vi "Dashboard Main.vi"() -> ()   [LabVIEW 2012]
uses:
  <vilib>/event_ctls.llb/eventvkey.ctl
  <vilib>/Utility/config.llb/Read Key (String).vi
  <vilib>/Utility/config.llb/Read Key (I32).vi
  <vilib>/Utility/config.llb/Write Key (String).vi
  <vilib>/Utility/config.llb/Write Key (I32).vi
  <vilib>/Utility/config.llb/NI_LVConfig.lvlib
panel:
  out "Battery Value":dbl(slide) scale=0.0..14.0 scale format="%#_2e"
  out "Battery":sgl(graph)
  in  "Camera Settings":T1={"Frate Rate"=30, "Compression"=30, "Size"=1} {"Frate Rate" scale=1.0..30.0; "Size" items=["640x480", "320x240", "160x120"]}
  out "Mode":T2(ring)=enum."Auto Disabled"
  out "Camera IP":string
  out "JS1 Z":dbl(slide) scale=-1.0..1.0 scale format="%#_2e"
  out "JS2 Z":dbl(slide) scale=-1.0..1.0 scale format="%#_2e"
  out "Joystick 1":cluster{"X":dbl, "Y":dbl}[](graph)
  out "Joystick 2":cluster{"X":dbl, "Y":dbl}[](graph)
  out "JS Buttons 1":T3
  out "JS Buttons 2":T3
  out "MotorSlide4":dbl(slide) scale=-1.0..1.0 scale format="%#_2e"
  out "MotorSlide3":dbl(slide) scale=-1.0..1.0 scale format="%#_2e"
  out "MotorSlide2":dbl(slide) scale=-1.0..1.0 scale format="%#_2e"
  out "MotorName3":string="Front Left"
  out "MotorName4":string="Front Right"
  out "MotorName1":string="Rear Left"
  out "MotorName2":string="Rear Right"
  out "MotorChart4":dbl(graph)
  out "MotorChart3":dbl(graph)
  out "MotorChart2":dbl(graph)
  out "MotorSlide1":dbl(slide) scale=-1.0..1.0 scale format="%#_2e"
  out "MotorChart1":dbl(graph)
  out "Robot IP":string
  in  "Dashboard Tab":T4(tab)
  in  "Disable Autonomous":bool
  out "Arm Hook Sensor":bool
  out "Arm Encoder":dbl(knob) scale=0.0..100.0
  in  "notes":string
  out "Right Hook Sensor":bool
  out "Left Hook Sensor":bool
  out "Encoder Set":bool
  out "Arm Limit":bool
  in  "Y-Throttle":dbl(slide)=1.0 min=0.0 max=1.0 step=0.1 scale=0.0..1.0
  in  "X-Throttle":dbl(slide)=1.0 min=0.0 max=1.0 step=0.1 scale=0.0..1.0
  in  "Dev Notes":string
  in  "Robot Subsystems":enum32{"Drive", "Arm", "Sensors", "Hotkeys"}(tab)
  out "Left Wheel Encoder":dbl
  out "Right Wheel Encoder":dbl
  in  "Override Limit":bool
  out "Right Ultrasonic PWM":dbl(slide) scale=0.0..100.0
  out "Gyro":dbl(knob) scale=-180.0..180.0
  out "Left Ultrasonic PWM":dbl(slide) scale=0.0..100.0
  out "Hotkey Step":dbl
  out "Arm Preset":dbl
  in  "Current Hotkey":string
  out "Hotkey Running?":bool
  in  "Sim":bool=TRUE
  in  "Slider":dbl(slide) scale=0.0..100.0 scale format="%#_3g"
  in  "On/Off":bool caption="Solenoid"
  in  "Test Name":u16(ring) items=["Select the test to run...", "Example Test", "-------------------------------", "List of tests is built in robot code.", "Replace with your own automated tests."]
  in  "Test Tree":string(tree)
  in  "Motor":cluster{"Value":dbl, "Enable":bool} {"Value" scale=-1.0..1.0 scale format="%#_3g"}
  out "Progress":T5 {"Test Progress" scale=0.0..100.0}
  in  "Rev/Fwd":cluster{"Forward":bool, "Reverse":bool}
  in  "Ring":u16(ring) items=["Auto", "Fixed indoor", "Fixed outdoor 1", "Fixed outdoor 2", "Fixed fluorescent 1", "Fixed fluorescent 2", "Hold current"]
  in  "Listbox":i32(listbox)
  in  "Viewer":T6(tab)
  out "Mbps":dbl format="%#.1g"
  in  "Enable":bool
  in  "DB Camera Config":bool
  out "Mbps":bool
  out "fps":dbl format="%#.1g"
  out "Image Error Message":string="Timeout in Camera Communications"
  out "Camera Image":T7(plugin-control)
  out "Buttons 1":cluster{"1":bool, "2":bool, "3":bool}
  out "Kinect 1":cluster{"X":dbl, "Y":dbl, "Z":dbl} {"X" scale=1.0..-1.0; "Y" scale=1.0..-1.0; "Z" scale=1.0..-1.0}
  out "Buttons 2":cluster{"1":bool, "2":bool, "3":bool}
  out "Kinect 2":cluster{"X":dbl, "Y":dbl, "Z":dbl} {"X" scale=1.0..-1.0; "Y" scale=1.0..-1.0; "Z" scale=1.0..-1.0}
  out "Version":string
  out "Skeleton Picture":picture
  out "Players":i8
  out "Tree":string(tree)
  # "Drive & Motors"
  # "Robot IP:"
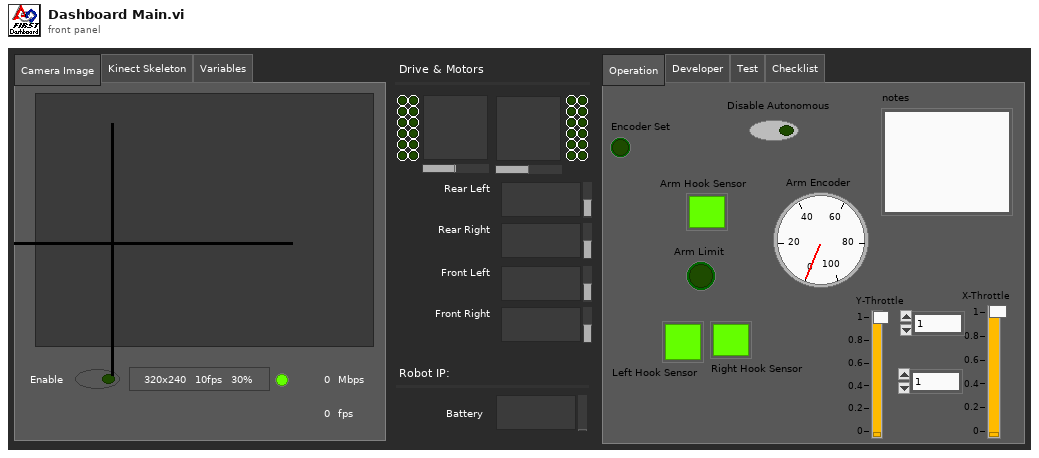
[diagram p1: front panel]
types:
  T1 = cluster{"Frate Rate":i32, "Compression":i32, "Size":u16}
  T2 = enum8{"Tele-Op Disabled", "Tele-Op Enabled", "Auto Disabled", "Auto Enabled", "Test Disabled", "Test Enabled", ""}
  T3 = cluster{bool, bool, bool, bool, bool, bool, bool, bool, bool, bool, bool, bool}
  T4 = enum32{"Operation", "Developer", "Test", "Checklist"}
  T5 = cluster{"Test Progress":u8, "Test Progress Text":string}
  T6 = enum32{"Camera Image", "Kinect Skeleton", "Variables"}
  T7 = typedef "IMAQ Image.ctl" = refnum<image>
  T8 = typedef "Image Type" = u32
  T9 = typedef "LVBoundsTypeDef.ctl" = cluster{"Width":u32, "Height":u32}
  T10 = typedef "SkeletonTrackState.ctl" = enum32{"NotTracked", "PositionOnly", "Tracked"}
  T11 = cluster{"TrackingState":u8[], "Position":cluster{"x":sgl, "y":sgl, "z":sgl}, cluster{"x":sgl, "y":sgl, "z":sgl, sgl}[], "TrackState":T10}
  T12 = cluster{cluster{"ScaledToPercentRange":dbl, "ScaledToPercentRange":dbl, "ScaledToPercentRange":dbl}, cluster{bool, bool, bool}}[]
  T13 = cluster{cluster{"ScaledToPercentRange":dbl, "ScaledToPercentRange":dbl, "ScaledToPercentRange":dbl}, cluster{bool, bool, bool}}
  T14 = cluster{"ScaledToPercentRange":dbl, "ScaledToPercentRange":dbl, "ScaledToPercentRange":dbl}
  T15 = typedef "LVRectTypeDef.ctl" = cluster{"Left":i16, "Top":i16, "Right":i16, "Bottom":i16}
  T16 = cluster{"Competition mode":bool, "Robot Link":bool, "Autonomous":bool, "Enabled":bool, "E-Stop":bool, "Simulated":bool, "TestMode":bool, "Docked Window":bool}
  T17 = cluster{"Boolean Array[0]":bool, "Boolean Array[1]":bool, "Boolean Array[2]":bool, "Boolean Array[3]":bool, "Boolean Array[4]":bool, "Boolean Array[5]":bool, "Boolean Array[6]":bool, "Boolean Array[7]":bool, "Boolean Array[8]":bool, "Boolean Array[9]":bool, "Boolean Array[10]":bool, "Boolean Array[11]":bool}
  T18 = typedef "NI_LVConfig.lvlib/Config Data RefNum.ctl" = refnum<k1>
  T19 = typedef "eventvkey.ctl" = enum16{"ASCII", "Enter", "Return", "Shift", "Ctrl", "Alt", "Cmd", "Opt", "Caps", "NumLock", "Clear", "Break", "Up", "Down", "Left", "Right", "Insert", "Delete", "Home", "End", "PageUp", "PageDown", "Escape", "Help", "Pause", "ScrollLock", "F1", "F2", "F3", "F4", "F5", "F6", "F7", "F8", "F9", "F10", "F11", "F12", "F13", "F14", "F15", "F16", "F17", "F18", "F19", "F20", "F21", "F22", "F23", "F24", "Play", "VolumeUp", "VolumeDown", "Mute", "Two Byte Char"}
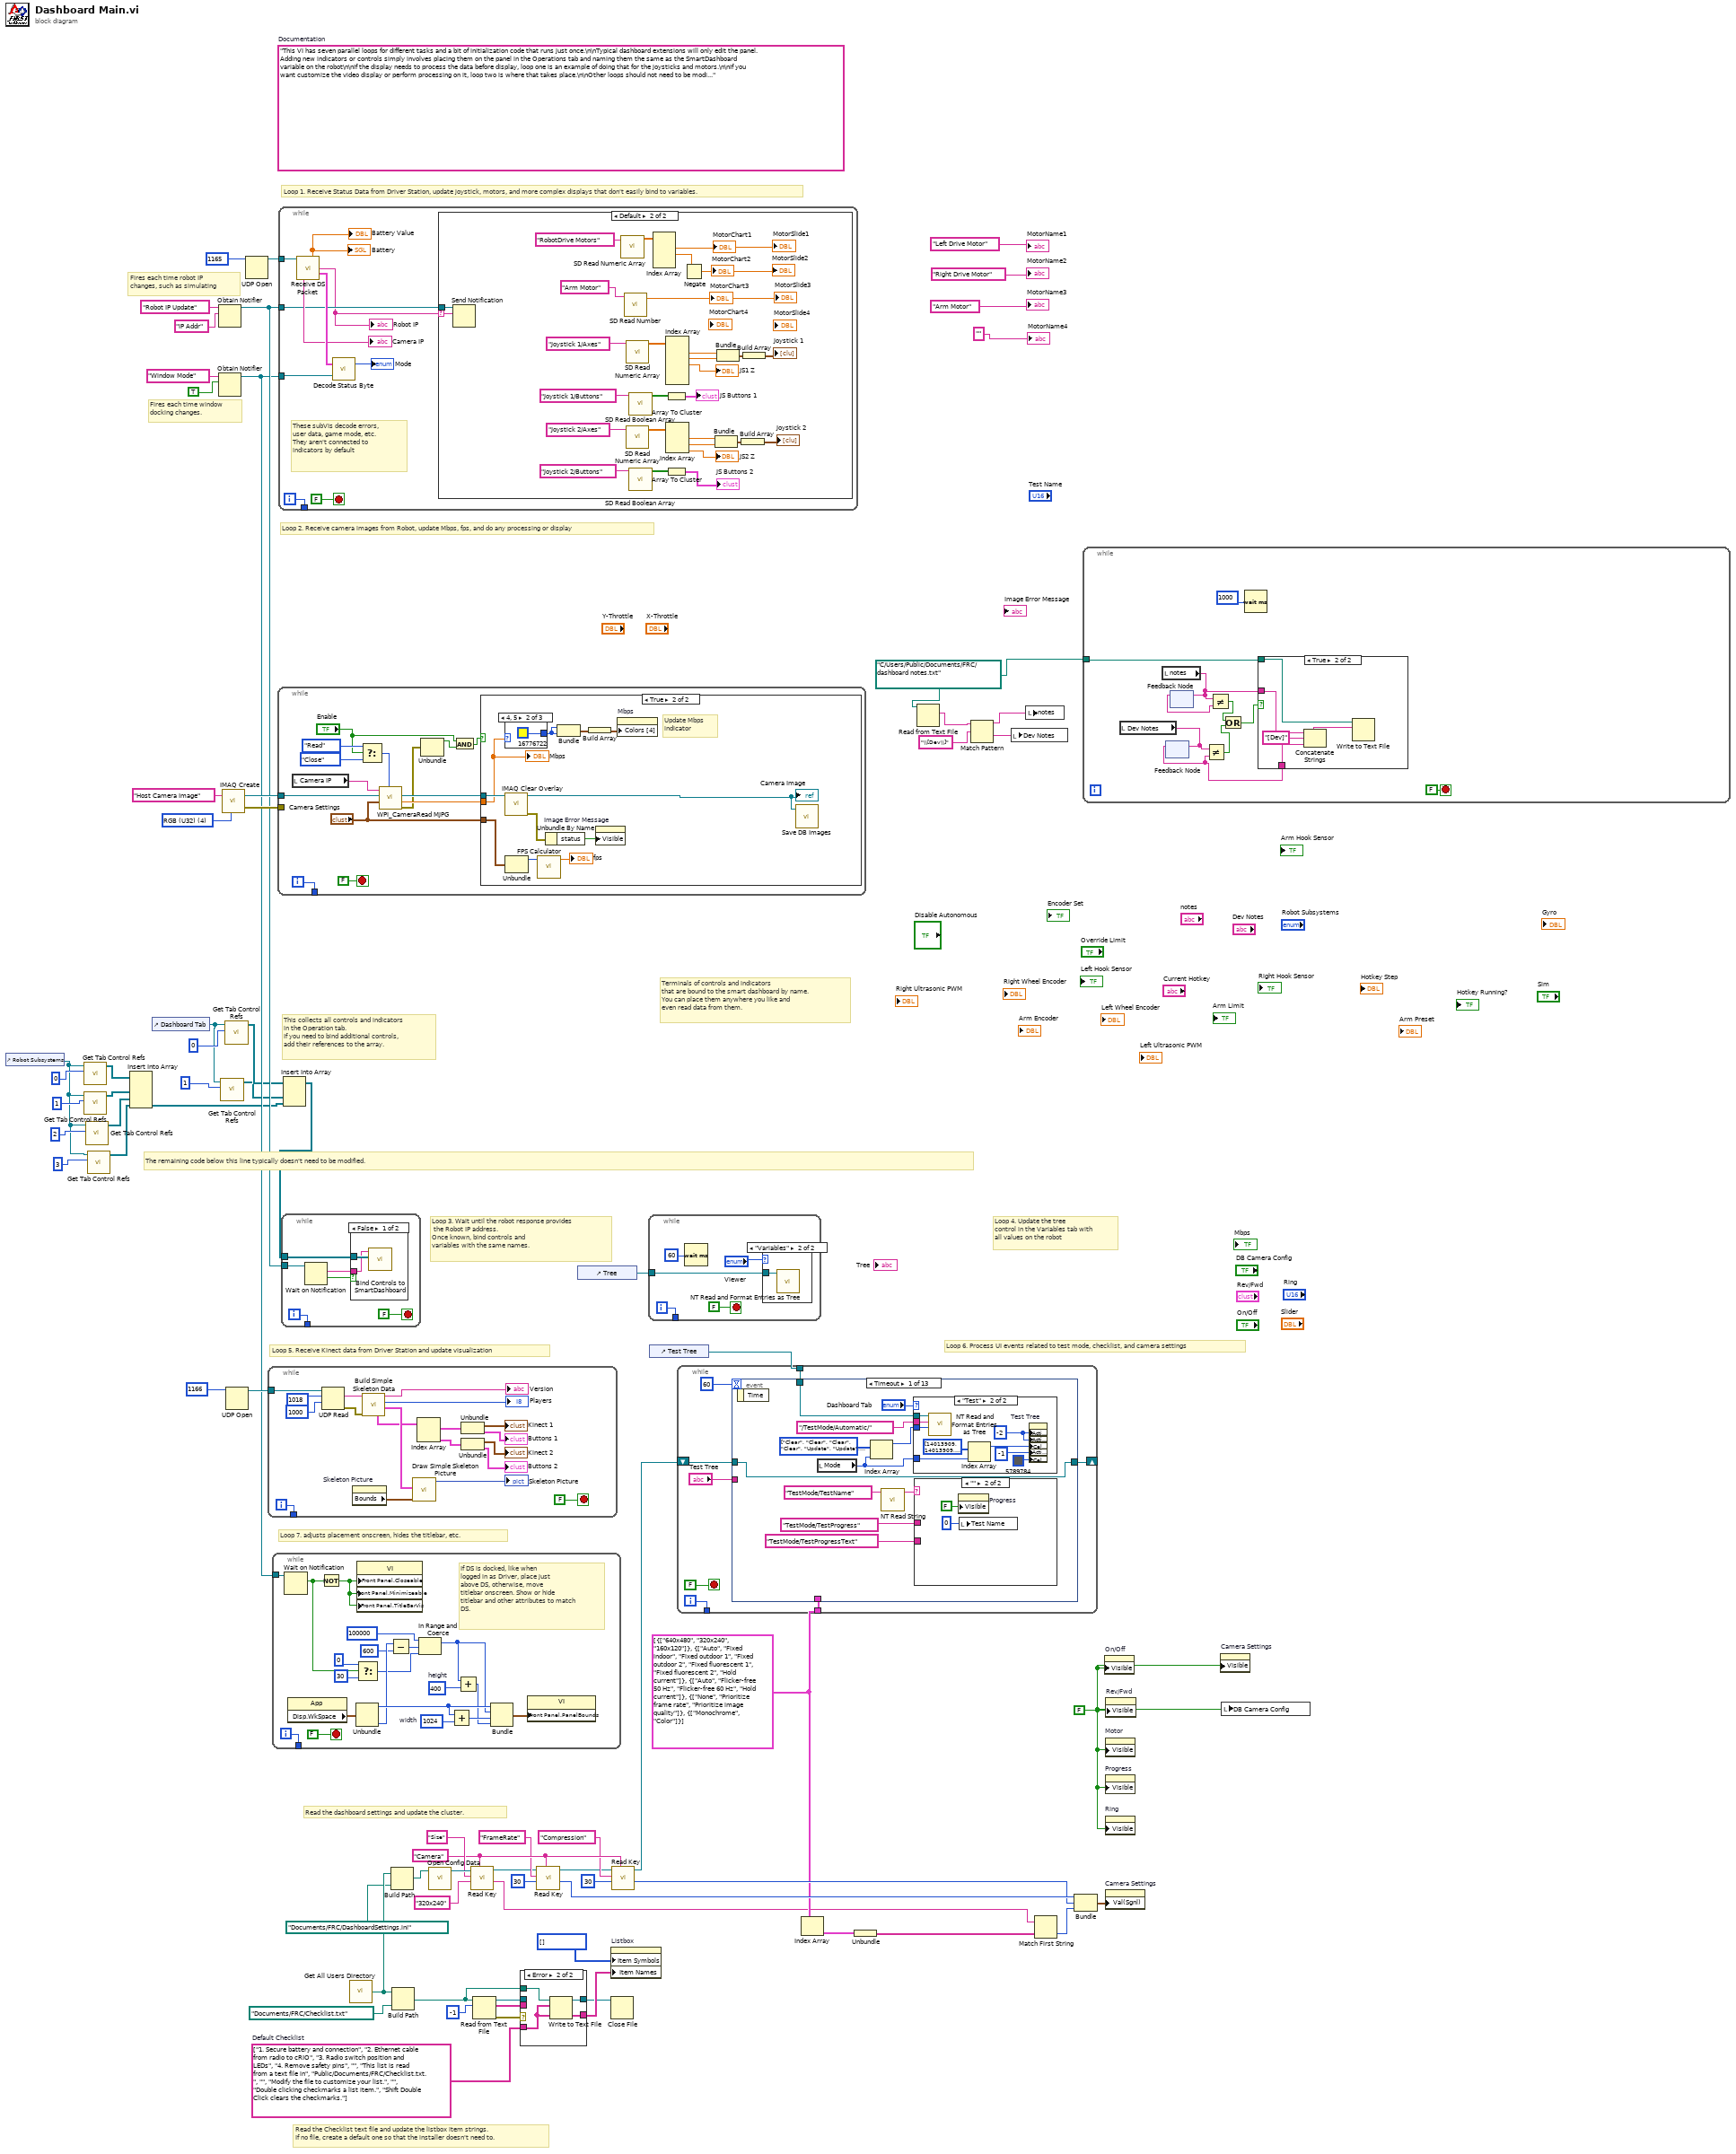
[diagram p0: block diagram]
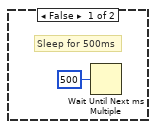
[diagram p4: hidden frame]
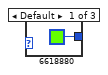
[diagram p5: hidden frame]
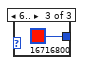
[diagram p6: hidden frame]
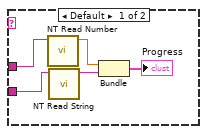
[diagram p9: hidden frame]
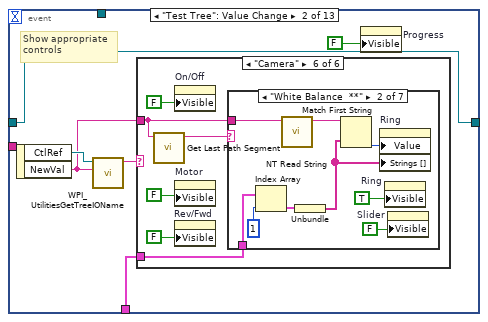
[diagram p10: hidden frame]
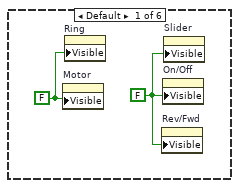
[diagram p11: hidden frame]
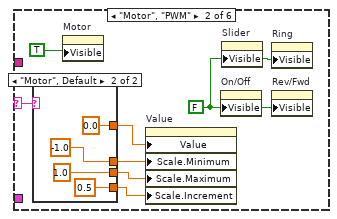
[diagram p12: hidden frame]
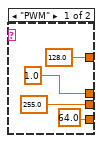
[diagram p13: hidden frame]
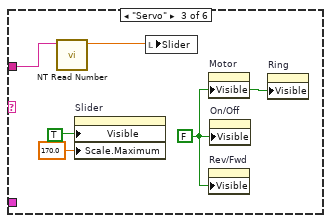
[diagram p14: hidden frame]
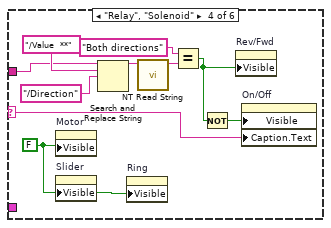
[diagram p15: hidden frame]
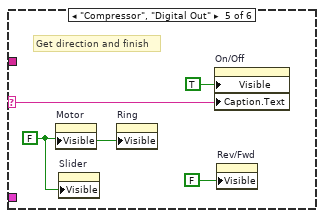
[diagram p16: hidden frame]
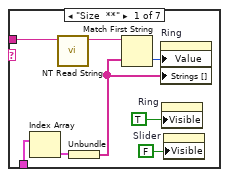
[diagram p17: hidden frame]
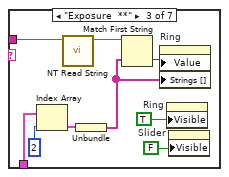
[diagram p18: hidden frame]
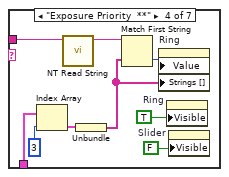
[diagram p19: hidden frame]
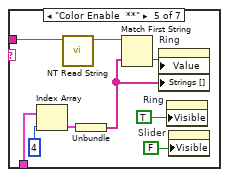
[diagram p20: hidden frame]
diagram:
  w15 = path "C:/Users/Public/Documents/FRC/dashboard notes.txt"
  w46 = "Camera"
  w38 = cluster{string[]}[] [{["640x480", "320x240", "160x120"]}, {["Auto", "Fixed indoor", "Fixed outdoor 1", "Fixed outdoor 2", "Fixed fluorescent 1", "Fixed fluorescent 2", "Hold current"]}, {["Auto", "Flicker-free 50 Hz", "Flicker-free 60 Hz", "Hold current"]}, {["None", "Prioritize frame rate", "Prioritize image quality"]}, {["Monochrome", "Color"]}]
  w54 = string[] ["1. Secure battery and connection", "2. Ethernet cable from radio to cRIO", "3. Radio switch position and LEDs", "4. Remove safety pins", "", "This list is read from a text file in", "Public/Documents/FRC/Checklist.txt.", "", "Modify the file to customize your list.", "", "Double clicking checkmarks a list item.", "Shift Double Click clears the checkmarks."]  # Default Checklist
  w52 = FALSE ("Visible")
  (unwired) "This VI has seven parallel loops for different tasks and a bit of initialization code that runs just once.\n\nTypical dashboard extensions will only edit the panel. Adding new indicators or controls simply involves placing them on the panel in the Operations tab and naming them the same as the SmartDashboard variable on the robot\n\nIf the display needs to process the data before display, loop one is an example of doing that for the joysticks and motors.\n\nIf you want customize the video display or perform processing on it, loop two is where that takes place.\n\nOther loops should not need to be modified. They are pretty standard, and document the task they perform."  # Documentation
  w72 = T8 4 items=["Grayscale (U8)", "Grayscale (I16)", "Grayscale (SGL)", "Complex (CSG)", "RGB (U32)", "HSL (U32)", "RGB (U64)"] ("Image Type")
  # "Fires each time robot IP\nchanges, such as simulating"
  # "Fires each time window\ndocking changes."
  # "Read the Checklist text file and update the listbox item strings.\nIf no file, create a default one so that the installer doesn't need to."
  # "This collects all controls and indicators\nin the Operation tab.\nIf you need to bind additional controls,\nadd their references to the array."
  # "The remaining code below this line typically doesn't need to be modified."
  # "Loop 6. Process UI events related to test mode, checklist, and camera settings"
  # "Read the dashboard settings and update the cluster."
  # "Terminals of controls and indicators\nthat are bound to the smart dashboard by name.\nYou can place them anywhere you like and\neven read data from them."
  # "Loop 4. Update the tree\ncontrol in the Variables tab with\nall values on the robot"
  # "Loop 3. Wait until the robot response provides\n the Robot IP address.\nOnce known, bind controls and\nvariables with the same names."
  # "Loop 5. Receive Kinect data from Driver Station and update visualization"
  # "Loop 7. adjusts placement onscreen, hides the titlebar, etc."
  # "Loop 1. Receive Status Data from Driver Station, update joystick, motors, and more complex displays that don't easily bind to variables."
  # "Loop 2. Receive camera images from Robot, update Mbps, fps, and do any processing or display"
  n1 = control-ref of="Robot Subsystems"() -> (w4:refnum<vi>)
  n2 = call <vilib>:"Get Tab Control Refs.vi"("Page Index"=0, "TabControl in"=w4) -> ("ControlsOnPage"=w8:refnum<vi>[])  [unwired: 9 in]
  n3 = call <vilib>:"Get Tab Control Refs.vi"("Page Index"=1, "TabControl in"=w4) -> ("ControlsOnPage"=w3:refnum<vi>[])  [unwired: 9 in]
  n4 = call <vilib>:"Get Tab Control Refs.vi"("Page Index"=2, "TabControl in"=w4) -> ("ControlsOnPage"=w2:refnum<vi>[])  [unwired: 9 in]
  n5 = call <vilib>:"Get Tab Control Refs.vi"("Page Index"=3, "TabControl in"=w4) -> ("ControlsOnPage"=w1:refnum<vi>[])  [unwired: 9 in]
  n6 = Insert Into Array(array=w8, new element #1=w3, new element #2=w2, new element #3=w1) -> (w9:refnum<vi>[])  [unwired: 1 in]
  n7 = control-ref of="Dashboard Tab"() -> (w19:refnum<vi>)
  n8 = Obtain Notifier(name (unnamed)="Robot IP Update", notification data type="IP Addr" ("name (unnamed)")) -> (notifier out=w64:refnum<notifier>)  [unwired: 2 in, 2 out]
  n9 = Obtain Notifier(name (unnamed)="Window Mode", notification data type=TRUE) -> (notifier out=w58:refnum<notifier>)  [unwired: 2 in, 2 out]
  n10 = call <vilib>:"Get Tab Control Refs.vi"("Page Index"=1, "TabControl in"=w19) -> ("ControlsOnPage"=w17:refnum<vi>[])  [unwired: 9 in]
  n11 = call "IMAQ Create"("Image Name"="Host Camera Image", "Image Type"=w72) -> ("New Image"=w70:T7, "error out"=w69:errorcluster)  [unwired: 2 in, 1 out]
  n12 = call <vilib>:"Get Tab Control Refs.vi"("Page Index"=0, "TabControl in"=w19) -> ("ControlsOnPage"=w21:refnum<vi>[])  [unwired: 9 in]
  n13 = UDP Open(11:u16 1166 ("port")) -> (port=w67:refnum<k16>)  [unwired: 2 in, 4 out]
  n14 = UDP Open(11:u16 1165 ("port")) -> (port=w73:refnum<k16>)  [unwired: 2 in, 4 out]
  n15 = while {
    tunnel: w67 -> [w91]
    tunnel: [w76] -> _
    i -> [w76]
    stop <- FALSE stop-if-true
    n16 = UDP Read(connection ID=w91, max size (548)=1018 ("bytes to read"), timeout ms (25000)=1000) -> (data out=w85:string, error out=w75:errorcluster)  [unwired: 1 in, 3 out]
    n17 = property on="Skeleton Picture" class="Pict"() -> ("Bounds"=w87:T9)  [unwired: 2 in, 2 out]
    n18 = call "Build Simple Skeleton Data.vi"("error in (no error)"=w75, "data in"=w85) -> ("Skeleton Data"=w86:T11, "NumPlayers"=→"Players":i8, "Version String"=→"Version":string, "Simple Joystick Info"=w83:T12)  [unwired: 5 in, 1 out]
    n19 = call "Draw Simple Skeleton Picture.vi"("Bounds"=w87, "Simple Skeleton"=w86) -> ("new picture out"=→"Skeleton Picture":picture)  [unwired: 9 in]
    n20 = Index Array(array=w83) -> (element #1=w82:T13, element #2=w81:T13)  [unwired: 2 in]
    n21 = Unbundle(w82) -> (→"Kinect 1":T14, →"Buttons 1":cluster{bool, bool, bool})
    n22 = Unbundle(w81) -> (→"Kinect 2":T14, →"Buttons 2":cluster{bool, bool, bool})
  }
  n23 = while {
    tunnel: w58 -> [w112]
    tunnel: [w110] -> _
    i -> [w110]
    stop <- FALSE stop-if-true
    w102 = 1024  # width
    w105 = 400  # height
    # "If DS is docked, like when\nlogged in as Driver, place just\nabove DS, otherwise, move\ntitlebar onscreen. Show or hide\ntitlebar and other attributes to match\nDS."
    n24 = Wait on Notification(notifier=w112) -> (notification=w97:bool)  [unwired: 3 in, 3 out]
    n25 = property class="App"() -> ("Disp.WkSpace"=w108:T15)  [unwired: 2 in, 2 out]
    n26 = Not(x=w97) -> (.not. x?=w111:bool)
    n27 = Unbundle(w108) -> ("Left"=w106:i16, "Bottom"=w103:i16)  [unwired: 2 out]
    n28 = Select(t=0, s=w97, f=30) -> (s? t:f=w96:i32)
    n29 = property class="VI"("Front Panel.Closeable"=w111, "Front Panel.Minimizeable"=w111, "Front Panel.TitleBarVis"=w111) -> ()  [unwired: 2 in, 2 out]
    n30 = Subtract(x=w103, y=600) -> (x-y=w100:i32)
    n31 = In Range and Coerce(upper limit=100000, x=w100, lower limit=w96) -> (coerced(x)=w94:i32)  [unwired: 1 out]
    n32 = Add(x=w106, y=w102) -> (x+y=w107:i32)
    n33 = Add(x=w94, y=w105) -> (x+y=w104:i32)
    n34 = Bundle("Left"=w106, w94, w107, w104) -> (w109:cluster{"Left":i16, i32, i32, i32})  [unwired: 1 out]
    n35 = property class="VI"("Front Panel.PanelBounds"=w109) -> ()  [unwired: 2 in, 2 out]
  }
  n36 = while {
    tunnel: w70 -> [w123]
    tunnel: w69 -> [_]
    tunnel: [w126] -> _
    i -> [w126]
    stop <- FALSE stop-if-true
    n37 = local read "Camera IP"() -> (w125:string)
    n38 = Select(t=enum16{"Read", "Reopen", "Close"}."Read" ("Operation"), s="Enable", f=enum16{"Read", "Reopen", "Close"}."Close" ("Operation")) -> (s? t:f=w118:enum16{"Read", "Reopen", "Close"})
    n39 = call <vilib>:"WPI_CameraRead MJPG.vi"("Operation"=w118, "Camera Settings"="Camera Settings", "Image"=w123, "address"=w125) -> ("error out"=w117:errorcluster, "Bandwidth (kbps)"=w121:dbl, "Image Out"=w122:T7)  [unwired: 5 in]
    n40 = Unbundle(w117) -> ("status"=w114:bool)  [unwired: 2 out]
    n41 = And(x="Enable", y=w114) -> (x .and. y?=w116:bool)
    n42 = case shown="True" w116 {
      tunnel: "Camera Settings" -> [_ w131]
      tunnel: w122 -> [_ w134]
      tunnel: w121 -> [_ w133]
      frame False {
        # "Sleep for 500ms"
        n43 = Wait Until Next ms Multiple(millisecond multiple=u32 500) -> ()  [unwired: 1 out]
      }
      frame True {
        # "Update Mbps\nindicator"
        n44 = call "IMAQ Clear Overlay"("Image"=w134) -> ("error out"=w138:errorcluster, "Image Out"=w129:T7)  [unwired: 2 in, 7 out]
        "Camera Image" <- w129
        n45 = case shown="4, 5" w133 {
          tunnel: [u32 6618880 ("Color Box") u32 16776722 ("Color Box") u32 16716800 ("Color Box")] -> w135
          frame Default {
          }
          frame 4, 5 {
          }
          frame 6.. {
          }
        }
        n46 = Unbundle(w131) -> ("Frate Rate"=w130:i32)  [unwired: 2 out]
        n47 = call "FPS Calculator.vi"("Average Count"=w130) -> ("fps"=→"fps":dbl)  [unwired: 10 in]
        n48 = Unbundle By Name(w138) -> ("status"=w139:bool)
        n49 = Bundle("Color Box"=w135, "Color Box"=w135) -> (w137:cluster{"Color Box":u32, "Color Box":u32})  [unwired: 1 out]
        n50 = Build Array(w137) -> (w136:cluster{"Color Box":u32, "Color Box":u32}[])
        n51 = property on="Image Error Message" class="Str"("Visible"=w139) -> ()  [unwired: 2 in, 2 out]
        n52 = property on="Mbps" class="Bool (strict)"("Colors [4]"=w136) -> ()  [unwired: 2 in, 2 out]
        n53 = call "Save DB Images.vi"("Image"=w129) -> ()  [unwired: 2 in, 1 out]
        "Mbps" <- w133
      }
    }
  }
  n54 = while {
    tunnel: w73 -> [w150]
    tunnel: w64 -> [w144]
    tunnel: w58 -> [w148]
    tunnel: [w145] -> _
    i -> [w145]
    stop <- FALSE stop-if-true
    # "These subVIs decode errors, user data, game mode, etc.\nThey aren't connected to indicators by default"
    n55 = call "Receive DS Packet.vi"("Recv Socket"=w150) -> ("Battery"=→"Battery" →"Battery Value":sgl, "Robot IP Address"=w143:string, "Status"=w151:T16, "Camera IP Address"=→"Camera IP":string)  [unwired: 1 in, 10 out]
    "Robot IP" <- w143
    n56 = call "Decode Status Byte.vi"("Window Mode Notifier"=w148, "Status"=w151) -> ("Mode"=→"Mode":T2)  [unwired: 1 out]
    n57 = case shown="Default" w143 {
      selector: w143 -> [_ w158]
      tunnel: w144 -> [_ w159]
      frame "0.0.0.0" {
        # "Robot not responding, don't poll the variables"
      }
      frame Default {
        n58 = Send Notification(notification=w158, notifier=w159) -> ()  [unwired: 1 in, 2 out]
        n59 = call <vilib>:"SD Read Numeric Array.vi"("Name"="RobotDrive Motors") -> ("Numeric Array"=w178:dbl[])  [unwired: 8 in, 2 out]
        n60 = call <vilib>:"SD Read Number.vi"("Name"="Arm Motor") -> ("Numeric"=→"MotorChart3" →"MotorSlide3":dbl)  [unwired: 8 in, 2 out]
        n61 = call <vilib>:"SD Read Numeric Array.vi"("Name"="Joystick 1/Axes") -> ("Numeric Array"=w174:dbl[])  [unwired: 8 in, 2 out]
        n62 = call <vilib>:"SD Read Numeric Array.vi"("Name"="Joystick 2/Axes") -> ("Numeric Array"=w169:dbl[])  [unwired: 8 in, 2 out]
        n63 = call <vilib>:"SD Read Boolean Array.vi"("Name"="Joystick 1/Buttons") -> ("Boolean Array"=w176:bool[])  [unwired: 8 in, 2 out]
        n64 = call <vilib>:"SD Read Boolean Array.vi"("Name"="Joystick 2/Buttons") -> ("Boolean Array"=w168:bool[])  [unwired: 8 in, 2 out]
        n65 = Index Array(array=w178) -> (element #1=→"MotorChart1" →"MotorSlide1":dbl, element #2=w154:dbl)  [unwired: 4 in, 2 out]
        n66 = Array To Cluster(array=w176) -> (cluster=→"JS Buttons 1":T17)
        n67 = Array To Cluster(array=w168) -> (cluster=→"JS Buttons 2":T17)
        n68 = Index Array(array=w174) -> (element #1=w172:dbl, element #2=w173:dbl, element #3=→"JS1 Z":dbl)  [unwired: 6 in, 3 out]
        n69 = Index Array(array=w169) -> (element #1=w164:dbl, element #2=w163:dbl, element #3=→"JS2 Z":dbl)  [unwired: 3 in]
        n70 = Negate(x=w154) -> (-x=→"MotorSlide2" →"MotorChart2":dbl)
        n71 = Bundle("Numeric"=w164, "Numeric"=w163) -> (w165:cluster{"Numeric":dbl, "Numeric":dbl})  [unwired: 1 in]
        n72 = Bundle("Numeric"=w172, "Numeric"=w173) -> (w171:cluster{"Numeric":dbl, "Numeric":dbl})  [unwired: 1 in]
        n73 = Build Array(w165) -> (→"Joystick 2":cluster{"Numeric":dbl, "Numeric":dbl}[])
        n74 = Build Array(w171) -> (→"Joystick 1":cluster{"Numeric":dbl, "Numeric":dbl}[])
      }
    }
  }
  n75 = Insert Into Array(array=w21, new element #1=w17, new element #2=w9) -> (w20:refnum<vi>[])  [unwired: 1 in]
  n76 = while {
    tunnel: w20 -> [w187]
    tunnel: w64 -> [w184]
    tunnel: [w182] -> _
    i -> [w182]
    stop <- FALSE stop-if-true
    n77 = Wait on Notification(notifier=w184) -> (notification=w183:string, timed out?=w185:bool)  [unwired: 3 in, 2 out]
    n78 = case shown="False" w185 {
      tunnel: w187 -> [w189 _]
      tunnel: w183 -> [w188 _]
      frame False {
        n79 = call <vilib>:"Bind Controls to SmartDashboard.vi"("Bound Control Refs"=w189, "Server IP Address"=w188) -> ()  [unwired: 10 in]
      }
      frame True {
      }
    }
  }
  n80 = call "Get All Users Directory.vi"() -> ("All User Path"=w51:path)
  n81 = Build Path(base path=w51, name or relative path=path "Documents/FRC/DashboardSettings.ini") -> (appended path=w50:path)
  n82 = Build Path(base path=w51, name or relative path=path "Documents/FRC/Checklist.txt") -> (appended path=w55:path)
  n83 = call <vilib>:"Open Config Data.vi"("configuration file path"=w50) -> ("refnum"=w49:T18)  [unwired: 8 in, 2 out]
  n84 = call-poly <vilib>:"Read Key.vi"("section"=w46, "default value"="320x240", "key"="Size", "refnum"=w49) -> ("value"=w36:string, "refnum out"=w31:T18)  [unwired: 2 in, 4 out]
  n85 = Read from Text File(file (use dialog)=w55, count=-1 ("timeout ms (25000)")) -> (refnum out=w33:refnum<file>, text=w56:string[], error out=w57:errorcluster)  [unwired: 2 in, 1 out]
  n86 = case shown="Error" w57 {
    tunnel: w56 -> [w191 _]
    tunnel: [w191 w193] -> w53
    tunnel: w54 -> [_ w193]
    tunnel: w55 -> [_ w194]
    tunnel: [w190 w192] -> w32
    tunnel: w33 -> [w190 _]
    frame No Error {
    }
    frame Error {
      n87 = Write to Text File(file (use dialog)=w194, text=w193) -> (refnum out=w192:refnum<file>)  [unwired: 2 in, 2 out]
    }
  }
  n88 = call-poly <vilib>:"Read Key.vi"("section"=w46, "default value"=30, "key"="FrameRate", "refnum"=w31) -> ("value"=w41:i32, "refnum out"=w30:T18)  [unwired: 1 in, 5 out]
  n89 = control-ref of="Tree"() -> (w27:refnum<vi>)
  n90 = property on="Listbox" class="LstBox (strict)"("Item Symbols"=i32[] [], "Item Names"=w53) -> ()  [unwired: 2 in, 2 out]
  n91 = Close File(refnum=w32) -> ()  [unwired: 1 in, 2 out]
  n92 = call-poly <vilib>:"Read Key.vi"("section"=w46, "default value"=30, "key"="Compression", "refnum"=w30) -> ("value"=w40:i32, "refnum out"=w28:T18)  [unwired: 1 in, 5 out]
  n93 = while {
    tunnel: [w196] -> _
    tunnel: w27 -> [w195]
    i -> [w196]
    stop <- FALSE stop-if-true
    n94 = Wait (ms)(milliseconds to wait=u32 60) -> ()  [unwired: 1 out]
    n95 = case shown="\"Variables\"" "Viewer" {
      tunnel: w195 -> [_ w200]
      frame Default {
      }
      frame "Variables" {
        n96 = call <vilib>:"NT Read and Format Entries as Tree.vi"("Tree Refnum"=w200) -> ()  [unwired: 9 in, 2 out]
      }
    }
  }
  n97 = control-ref of="Test Tree"() -> (w26:refnum<vi>)
  n98 = while {
    tunnel: w38 -> [w205]
    shift-right: [w204] -> _
    shift-left: w28 -> [w203]
    tunnel: [w202] -> _
    tunnel: w26 -> [w201]
    i -> [w202]
    stop <- FALSE stop-if-true
    n99 = event shown="[0] Timeout" {
      selector: _ -> [_ _ _ _ _ _ _ _ _ _ _ _ _]
      dyn-events: _ -> [_ _ _ _ _ _ _ _ _ _ _ _ _]
      timeout: u32 60 ("milliseconds to wait") -> [_ _ _ _ _ _ _ _ _ _ _ _ _]
      tunnel: w201 -> [w215 _ _ _ _ _ _ _ _ _ _ _ _]
      tunnel: "Test Tree" -> [_ _ _ _ _ _ _ _ w409 w417 w419 w423 w431]
      tunnel: w205 -> [_ w237 _ _ _ _ w373 w403 _ _ _ _ _]
      tunnel: [w209 w236 _ w339 w347 w359 w372 w396 w408 w415 w418 w422 w430] -> w204
      tunnel: w203 -> [w209 w236 _ w339 w347 w359 w371 w396 w408 w415 w418 w422 w430]
      event Timeout {
        w214 = enum16{"Update", "Clear"}[] [enum."Clear", enum."Clear", enum."Clear", enum."Clear", enum."Update", enum."Update", enum."Clear"] items=["Update", "Clear"]
        n100 = event-data() -> ()  [unwired: 1 in, 1 out]
        n101 = local read "Mode"() -> (w212:T2)
        n102 = Index Array(array=w214, index=w212) -> (element=w213:enum16{"Update", "Clear"})
        n103 = call <vilib>:"NT Read String.vi"("Name"="TestMode/TestName") -> ("String"=w218:string)  [unwired: 9 in, 1 out]
        n104 = case shown="\"Test\"" "Dashboard Tab" {
          tunnel: w215 -> [_ w228]
          tunnel: "/TestMode/Automatic/" ("Name Pattern") -> [_ w227]
          tunnel: w213 -> [_ w226]
          tunnel: w212 -> [_ w224]
          frame "Operation", Default {
          }
          frame "Test" {
            w223 = -2 ("Active Item:Row Number")
            n105 = call <vilib>:"NT Read and Format Entries as Tree.vi"("Operation"=w226, "Name Pattern"=w227, "Tree Refnum"=w228) -> ()  [unwired: 7 in, 2 out]
            n106 = Index Array(array=u32[] [14013909, 14013909, 14013909, 14013909, 14013909, 16777215, 14013909], index=w224) -> (element=w222:u32)
            n107 = property on="Test Tree" class="Tree (strict)"("Active Item Row Number"=w223, "ActiveColNum"=w223, "CellBG"=w222, "Active Item Row Number"=-1 ("Active Item:Row Number"), "CellBG"=u32 5789784 ("Color Box")) -> ()  [unwired: 2 in, 2 out]
          }
        }
        n108 = case shown="\"\"" w218 {
          tunnel: "TestMode/TestProgress" ("Name") -> [w230 _]
          tunnel: "TestMode/TestProgressText" ("Name") -> [w229 _]
          frame Default {
            n109 = call <vilib>:"NT Read Number.vi"("Name"=w230) -> ("Numeric"=w231:dbl)  [unwired: 9 in, 1 out]
            n110 = call <vilib>:"NT Read String.vi"("Name"=w229) -> ("String"=w232:string)  [unwired: 9 in, 1 out]
            n111 = Bundle("Numeric"=w231, "String"=w232) -> (→"Progress":cluster{"Numeric":dbl, "String":string})  [unwired: 1 in]
          }
          frame "" {
            n112 = property on="Progress" class="Clust (strict)"("Visible"=FALSE) -> ()  [unwired: 2 in, 2 out]
            n113 = local write "Test Name"(u16 0) -> ()
          }
        }
      }
      event "Test Tree": Value Change {
        # "Show appropriate\ncontrols"
        n114 = event-data() -> ("CtlRef"=w240:refnum<vi>, "NewVal"=w238:string)  [unwired: 1 in]
        n115 = call <vilib>:"WPI_UtilitiesGetTreeIOName.vi"("NewVal"=w238, "TreeControl in"=w240) -> ("I/O Name"=w241:string)  [unwired: 9 in]
        n116 = case shown="\"Camera\"" w241 {
          selector: w241 -> [_ w248 _ w266 w275 _]
          tunnel: w238 -> [_ _ w263 w265 _ w282]
          tunnel: w237 -> [_ _ _ _ _ w281]
          frame Default {
            w243 = FALSE ("Visible")
            w242 = FALSE ("Visible")
            n117 = property on="Motor" class="Clust (strict)"("Visible"=w242) -> ()  [unwired: 2 in, 2 out]
            n118 = property on="Ring" class="Ring (strict)"("Visible"=w242) -> ()  [unwired: 2 in, 2 out]
            n119 = property on="Rev/Fwd" class="Clust (strict)"("Visible"=w243) -> ()  [unwired: 2 in, 2 out]
            n120 = property on="On/Off" class="Bool (strict)"("Visible"=w243) -> ()  [unwired: 2 in, 2 out]
            n121 = property on="Slider" class="Slide (strict)"("Visible"=w243) -> ()  [unwired: 2 in, 2 out]
          }
          frame "Motor", "PWM" {
            w249 = FALSE ("Visible")
            n122 = case shown="\"Motor\", Default" w248 {
              tunnel: [1.0 ("Value") -1.0 ("Value")] -> w247
              tunnel: [255.0 ("Value") 1.0 ("Value")] -> w246
              tunnel: [128.0 ("Value") 0.0 ("Value")] -> w245
              tunnel: [64.0 ("Value") 0.5 ("Value")] -> w244
              frame "PWM" {
              }
              frame "Motor", Default {
              }
            }
            n123 = property on="Motor" class="Clust (strict)"("Visible"=TRUE) -> ()  [unwired: 2 in, 2 out]
            n124 = property on="Value" class="Slide (strict)"("Value"=w245, "Scale.Minimum"=w247, "Scale.Maximum"=w246, "Scale.Increment"=w244) -> ()  [unwired: 2 in, 2 out]
            n125 = property on="On/Off" class="Bool (strict)"("Visible"=w249) -> ()  [unwired: 2 in, 2 out]
            n126 = property on="Slider" class="Slide (strict)"("Visible"=w249) -> ()  [unwired: 2 in, 2 out]
            n127 = property on="Ring" class="Ring (strict)"("Visible"=w249) -> ()  [unwired: 2 in, 2 out]
            n128 = property on="Rev/Fwd" class="Clust (strict)"("Visible"=w249) -> ()  [unwired: 2 in, 2 out]
          }
          frame "Servo" {
            w261 = FALSE ("Visible")
            n129 = call <vilib>:"NT Read Number.vi"("Name"=w263) -> ("Numeric"=w262:dbl)  [unwired: 9 in, 1 out]
            n130 = property on="Slider" class="Slide (strict)"("Visible"=TRUE, "Scale.Maximum"=170.0 ("Scale.Range:Maximum")) -> ()  [unwired: 2 in, 2 out]
            n131 = local write "Slider"(w262) -> ()
            n132 = property on="Motor" class="Clust (strict)"("Visible"=w261) -> ()  [unwired: 2 in, 2 out]
            n133 = property on="Rev/Fwd" class="Clust (strict)"("Visible"=w261) -> ()  [unwired: 2 in, 2 out]
            n134 = property on="On/Off" class="Bool (strict)"("Visible"=w261) -> ()  [unwired: 2 in, 2 out]
            n135 = property on="Ring" class="Ring (strict)"("Visible"=w261) -> ()  [unwired: 2 in, 2 out]
          }
          frame "Relay", "Solenoid" {
            w264 = FALSE ("Visible")
            n136 = property on="Motor" class="Clust (strict)"("Visible"=w264) -> ()  [unwired: 2 in, 2 out]
            n137 = property on="Slider" class="Slide (strict)"("Visible"=w264) -> ()  [unwired: 2 in, 2 out]
            n138 = Search and Replace String(input string=w265, search string="/Value  **", replace string="/Direction") -> (result string=w271:string)  [unwired: 5 in, 3 out]
            n139 = property on="Ring" class="Ring (strict)"("Visible"=w264) -> ()  [unwired: 2 in, 2 out]
            n140 = call <vilib>:"NT Read String.vi"("Name"=w271) -> ("String"=w269:string)  [unwired: 9 in, 1 out]
            n141 = Equal?(x="Both directions", y=w269) -> (x = y?=w267:bool)
            n142 = Not(x=w267) -> (.not. x?=w268:bool)
            n143 = property on="Rev/Fwd" class="Clust (strict)"("Visible"=w267) -> ()  [unwired: 2 in, 2 out]
            n144 = property on="On/Off" class="Bool (strict)"("Visible"=w268, "Caption.Text"=w266) -> ()  [unwired: 2 in, 2 out]
          }
          frame "Compressor", "Digital Out" {
            w274 = FALSE ("Visible")
            # "Get direction and finish"
            n145 = property on="Motor" class="Clust (strict)"("Visible"=w274) -> ()  [unwired: 2 in, 2 out]
            n146 = property on="Slider" class="Slide (strict)"("Visible"=w274) -> ()  [unwired: 2 in, 2 out]
            n147 = property on="Ring" class="Ring (strict)"("Visible"=w274) -> ()  [unwired: 2 in, 2 out]
            n148 = property on="On/Off" class="Bool (strict)"("Visible"=TRUE, "Caption.Text"=w275) -> ()  [unwired: 2 in, 2 out]
            n149 = property on="Rev/Fwd" class="Clust (strict)"("Visible"=FALSE) -> ()  [unwired: 2 in, 2 out]
          }
          frame "Camera" {
            n150 = call <vilib>:"Get Last Path Segment.vi"("String in"=w282) -> ("String out"=w283:string)  [unwired: 10 in]
            n151 = property on="On/Off" class="Bool (strict)"("Visible"=FALSE) -> ()  [unwired: 2 in, 2 out]
            n152 = property on="Motor" class="Clust (strict)"("Visible"=FALSE) -> ()  [unwired: 2 in, 2 out]
            n153 = property on="Rev/Fwd" class="Clust (strict)"("Visible"=FALSE) -> ()  [unwired: 2 in, 2 out]
            n154 = case shown="\"White Balance  **\"" w283 {
              tunnel: w282 -> [w289 w298 w307 w316 w325 _ w331]
              tunnel: w281 -> [w287 w295 w304 w313 w322 _ _]
              frame "Size  **" {
                n155 = Index Array(array=w287) -> (element=w286:cluster{string[]})  [unwired: 1 in]
                n156 = call <vilib>:"NT Read String.vi"("Name"=w289) -> ("String"=w288:string)  [unwired: 9 in, 1 out]
                n157 = Unbundle(w286) -> (w284:string[])
                n158 = Match First String(2:w284, 3:w288) -> (0:w285:i32)  [unwired: 1 out]
                n159 = property on="Ring" class="Ring (strict)"("Value"=w285, "Strings []"=w284) -> ()  [unwired: 2 in, 2 out]
                n160 = property on="Ring" class="Ring (strict)"("Visible"=TRUE) -> ()  [unwired: 2 in, 2 out]
                n161 = property on="Slider" class="Slide (strict)"("Visible"=FALSE) -> ()  [unwired: 2 in, 2 out]
              }
              frame "White Balance  **" {
                n162 = Index Array(array=w295, index=1) -> (element=w296:cluster{string[]})
                n163 = call <vilib>:"NT Read String.vi"("Name"=w298) -> ("String"=w297:string)  [unwired: 9 in, 1 out]
                n164 = Unbundle(w296) -> (w293:string[])
                n165 = Match First String(2:w293, 3:w297) -> (0:w292:i32)  [unwired: 1 out]
                n166 = property on="Ring" class="Ring (strict)"("Value"=w292, "Strings []"=w293) -> ()  [unwired: 2 in, 2 out]
                n167 = property on="Ring" class="Ring (strict)"("Visible"=TRUE) -> ()  [unwired: 2 in, 2 out]
                n168 = property on="Slider" class="Slide (strict)"("Visible"=FALSE) -> ()  [unwired: 2 in, 2 out]
              }
              frame "Exposure  **" {
                n169 = Index Array(array=w304, index=2) -> (element=w305:cluster{string[]})
                n170 = call <vilib>:"NT Read String.vi"("Name"=w307) -> ("String"=w306:string)  [unwired: 9 in, 1 out]
                n171 = Unbundle(w305) -> (w301:string[])
                n172 = Match First String(2:w301, 3:w306) -> (0:w302:i32)  [unwired: 1 out]
                n173 = property on="Ring" class="Ring (strict)"("Value"=w302, "Strings []"=w301) -> ()  [unwired: 2 in, 2 out]
                n174 = property on="Ring" class="Ring (strict)"("Visible"=TRUE) -> ()  [unwired: 2 in, 2 out]
                n175 = property on="Slider" class="Slide (strict)"("Visible"=FALSE) -> ()  [unwired: 2 in, 2 out]
              }
              frame "Exposure Priority  **" {
                n176 = Index Array(array=w313, index=3) -> (element=w314:cluster{string[]})
                n177 = call <vilib>:"NT Read String.vi"("Name"=w316) -> ("String"=w315:string)  [unwired: 9 in, 1 out]
                n178 = Unbundle(w314) -> (w310:string[])
                n179 = Match First String(2:w310, 3:w315) -> (0:w311:i32)  [unwired: 1 out]
                n180 = property on="Ring" class="Ring (strict)"("Value"=w311, "Strings []"=w310) -> ()  [unwired: 2 in, 2 out]
                n181 = property on="Ring" class="Ring (strict)"("Visible"=TRUE) -> ()  [unwired: 2 in, 2 out]
                n182 = property on="Slider" class="Slide (strict)"("Visible"=FALSE) -> ()  [unwired: 2 in, 2 out]
              }
              frame "Color Enable  **" {
                n183 = Index Array(array=w322, index=4) -> (element=w323:cluster{string[]})
                n184 = call <vilib>:"NT Read String.vi"("Name"=w325) -> ("String"=w324:string)  [unwired: 9 in, 1 out]
                n185 = Unbundle(w323) -> (w319:string[])
                n186 = Match First String(2:w319, 3:w324) -> (0:w320:i32)  [unwired: 1 out]
                n187 = property on="Ring" class="Ring (strict)"("Value"=w320, "Strings []"=w319) -> ()  [unwired: 2 in, 2 out]
                n188 = property on="Ring" class="Ring (strict)"("Visible"=TRUE) -> ()  [unwired: 2 in, 2 out]
                n189 = property on="Slider" class="Slide (strict)"("Visible"=FALSE) -> ()  [unwired: 2 in, 2 out]
              }
              frame Default {
                n190 = property on="Ring" class="Ring (strict)"("Visible"=FALSE) -> ()  [unwired: 2 in, 2 out]
                n191 = property on="Slider" class="Slide (strict)"("Visible"=FALSE) -> ()  [unwired: 2 in, 2 out]
              }
              frame "Brightness  **", "Color Level  **", "Compression  **", "FPS  **", "Sharpness  **" {
                n192 = call <vilib>:"NT Read Number.vi"("Name"=w331) -> ("Numeric"=w330:dbl)  [unwired: 9 in, 1 out]
                n193 = local write "Slider"(w330) -> ()
                n194 = property on="Slider" class="Slide (strict)"("Visible"=TRUE, "Scale.Maximum"=100.0 ("Scale.Range:Maximum")) -> ()  [unwired: 2 in, 2 out]
                n195 = property on="Ring" class="Ring (strict)"("Visible"=FALSE) -> ()  [unwired: 2 in, 2 out]
              }
            }
          }
        }
        n196 = property on="Progress" class="Clust (strict)"("Visible"=FALSE) -> ()  [unwired: 2 in, 2 out]
      }
      event "Test Name": Mouse Enter {
        # "Populate the ring with the list of tests"
        n197 = event-data() -> ()  [unwired: 1 in, 1 out]
        n198 = call <vilib>:"NT Read String Array.vi"("Name"="TestMode/TestList") -> ("String Array"=w338:string[])  [unwired: 9 in, 1 out]
        n199 = Build Array (concatenate)("Select the test to run...", w338) -> (w337:string[])
        n200 = property on="Test Name" class="Ring (strict)"("Strings []"=w337) -> ()  [unwired: 2 in, 2 out]
      }
      event "Test Name": Value Change {
        w340 = FALSE ("Visible")
        # "Tell the robot the test name to run"
        n201 = event-data() -> ("NewVal"=w344:u16)  [unwired: 1 in]
        n202 = property on="Test Name" class="Ring (strict)"() -> ("Strings []"=w345:string[])  [unwired: 2 in, 2 out]
        n203 = local write "Progress"(T5 {"Test Progress"=0, "Test Progress Text"=""} ("Progress")) -> ()
        n204 = Index Array(array=w345, index=w344) -> (element=w343:string)
        n205 = call <vilib>:"NT Write String.vi"("String"=w343, "Name"="TestMode/TestName") -> ()  [unwired: 9 in, 1 out]
        n206 = property on="Progress" class="Clust (strict)"("Visible"=TRUE) -> ()  [unwired: 2 in, 2 out]
        n207 = property on="Motor" class="Clust (strict)"("Visible"=w340) -> ()  [unwired: 2 in, 2 out]
        n208 = property on="Slider" class="Slide (strict)"("Visible"=w340) -> ()  [unwired: 2 in, 2 out]
        n209 = property on="On/Off" class="Bool (strict)"("Visible"=w340) -> ()  [unwired: 2 in, 2 out]
        n210 = property on="Rev/Fwd" class="Clust (strict)"("Visible"=w340) -> ()  [unwired: 2 in, 2 out]
        n211 = property on="Ring" class="Ring (strict)"("Visible"=w340) -> ()  [unwired: 2 in, 2 out]
      }
      event "Listbox": Double Click {
        n212 = event-data() -> ("PlatMods.Shift"=w348:bool, "Row"=w350:i32)  [unwired: 1 in]
        n213 = case shown="False" w348 {
          tunnel: w350 -> [w354 _]
          tunnel: 1 -> [w353 _]
          frame False {
            n214 = property on="Listbox" class="LstBox (strict)"() -> ("Item Symbols"=w352:i32[])  [unwired: 2 in, 2 out]
            n215 = Replace Array Subset(array=w352, new element=w353, index=w354) -> (w351:i32[])
            n216 = property on="Listbox" class="LstBox (strict)"("Item Symbols"=w351) -> ()  [unwired: 2 in, 2 out]
          }
          frame True {
            w355 = 0 ("Top Row")
            n217 = property on="Listbox" class="LstBox (strict)"() -> ("Number of Rows"=w357:u32)  [unwired: 2 in, 2 out]
            n218 = Initialize Array(0, w357) -> (w356:i32[])
            n219 = property on="Listbox" class="LstBox (strict)"("Top Row"=w355, "Value"=w355, "Item Symbols"=w356) -> ()  [unwired: 2 in, 2 out]
          }
        }
      }
      event "Listbox": Key Down {
        n220 = event-data() -> ("VKey"=w361:T19)  [unwired: 1 in]
        n221 = case shown="\"Left\", \"Right\"" w361 {
          selector: w361 -> [w366 _]
          tunnel: eventvkey."Left" ("VKey") -> [w364 _]
          frame "Left", "Right" {
            n222 = Equal?(x=w364, y=w366) -> (x = y?=w365:bool)
            n223 = Select(t=0, s=w365, f=1) -> (s? t:f=w367:i32)
            n224 = property on="Listbox" class="LstBox (strict)"() -> ("Item Symbols"=w370:i32[])  [unwired: 2 in, 2 out]
            n225 = Replace Array Subset(array=w370, new element=w367, index="Listbox") -> (w369:i32[])
            n226 = property on="Listbox" class="LstBox (strict)"("Item Symbols"=w369) -> ()  [unwired: 2 in, 2 out]
          }
          frame Default {
          }
        }
      }
      event "DB Camera Config": Value Change {
        n227 = event-data() -> ("NewVal"=w374:bool)  [unwired: 1 in]
        n228 = case shown="False" w374 {
          tunnel: w373 -> [w383 _]
          tunnel: [w376 w394] -> w372
          tunnel: w371 -> [w375 w394]
          frame False {
            w390 = "Camera"
            w393 = FALSE ("Visible")
            n229 = local read "Camera Settings"() -> (w382:T1)
            n230 = Index Array(array=w383) -> (element=w386:cluster{string[]})  [unwired: 1 in]
            n231 = Unbundle(w382) -> ("Frate Rate"=w381:i32, "Compression"=w380:i32, "Size"=w384:u16)
            n232 = Unbundle(w386) -> (w385:string[])
            n233 = Index Array(array=w385, index=w384) -> (element=w379:string)
            n234 = call-poly <vilib>:"Write Key.vi"("section"=w390, "value"=w379, "key"="Size", "refnum"=w375) -> ("refnum out"=w392:T18)  [unwired: 2 in, 5 out]
            n235 = call-poly <vilib>:"Write Key.vi"("section"=w390, "value"=w381, "key"="FrameRate", "refnum"=w392) -> ("refnum out"=w391:T18)  [unwired: 1 in, 6 out]
            n236 = property on="Camera Settings" class="Clust (strict)"("Visible"=w393) -> ()  [unwired: 2 in, 2 out]
            n237 = local write "DB Camera Config"(w393) -> ()
            n238 = call-poly <vilib>:"Write Key.vi"("section"=w390, "value"=w380, "key"="Compression", "refnum"=w391) -> ("refnum out"=w377:T18)  [unwired: 1 in, 6 out]
            n239 = call <vilib>:"Close Config Data.vi"("refnum"=w377) -> ("file path"=w378:path)  [unwired: 2 in, 8 out]
            n240 = call <vilib>:"Open Config Data.vi"("configuration file path"=w378) -> ("refnum"=w376:T18)  [unwired: 8 in, 2 out]
          }
          frame True {
            n241 = property on="Camera Settings" class="Clust (strict)"("Visible"=TRUE) -> ()  [unwired: 2 in, 2 out]
          }
        }
      }
      event "Camera Settings": Value Change {
        n242 = event-data() -> ("NewVal"=w407:T1)  [unwired: 1 in]
        n243 = Index Array(array=w403) -> (element=w402:cluster{string[]})  [unwired: 1 in]
        n244 = Unbundle(w407) -> ("Frate Rate"=w398:i32, "Compression"=w397:i32, "Size"=w400:u16)
        n245 = Unbundle(w402) -> (w401:string[])
        n246 = Index Array(array=w401, index=w400) -> (element=w399:string)
        n247 = Format Into String(format string="%s   %dfps   %d%%", w399, w398, w397) -> (resulting string=w404:string)  [unwired: 2 in, 1 out]
        n248 = Build Array(w404) -> (w405:string[])
        n249 = property on="DB Camera Config" class="Bool (strict)"("Strings [4]"=w405) -> ()  [unwired: 2 in, 2 out]
      }
      event "Motor.Enable": Value Change {
        n250 = event-data() -> ("NewVal"=w413:bool)  [unwired: 1 in]
        n251 = Unbundle("Motor") -> ("Value"=w412:dbl)  [unwired: 1 out]
        n252 = Select(t=w412, s=w413, f=0.0) -> (s? t:f=w410:dbl)
        n253 = call <vilib>:"NT Write Number.vi"("Numeric"=w410, "Name"=w409) -> ()  [unwired: 9 in, 1 out]
      }
      event "Slider": Value Change {
        n254 = event-data() -> ("NewVal"=w416:dbl)  [unwired: 1 in]
        n255 = call <vilib>:"NT Write Number.vi"("Numeric"=w416, "Name"=w417) -> ()  [unwired: 9 in, 1 out]
      }
      event "On/Off": Value Change {
        n256 = event-data() -> ("NewVal"=w421:bool)  [unwired: 1 in]
        n257 = Boolean To (0,1)(Boolean=w421) -> (0, 1=w420:i16)
        n258 = call <vilib>:"NT Write Number.vi"("Numeric"=w420, "Name"=w419) -> ()  [unwired: 9 in, 1 out]
      }
      event "Rev/Fwd": Value Change {
        n259 = event-data() -> ("NewVal.Forward"=w429:bool, "NewVal.Reverse"=w428:bool)  [unwired: 1 in]
        n260 = Boolean To (0,1)(Boolean=w429) -> (0, 1=w425:i16)
        n261 = Boolean To (0,1)(Boolean=w428) -> (0, 1=w427:i16)
        n262 = Negate(x=w427) -> (-x=w426:i16)
        n263 = Add(x=w425, y=w426) -> (x+y=w424:i16)
        n264 = call <vilib>:"NT Write Number.vi"("Numeric"=w424, "Name"=w423) -> ()  [unwired: 9 in, 1 out]
      }
      event "Ring": Value Change {
        n265 = event-data() -> ("NewVal"=w433:u16)  [unwired: 1 in]
        n266 = property on="Ring" class="Ring (strict)"() -> ("Strings []"=w434:string[])  [unwired: 2 in, 2 out]
        n267 = Index Array(array=w434, index=w433) -> (element=w432:string)
        n268 = call <vilib>:"NT Write String.vi"("String"=w432, "Name"=w431) -> ()  [unwired: 9 in, 1 out]
      }
    }
  }
  n269 = Index Array(array=w38) -> (element=w39:cluster{string[]})  [unwired: 1 in]
  n270 = Unbundle(w39) -> (w37:string[])
  n271 = Read from Text File(file (use dialog)=w15) -> (text=w14:string)  [unwired: 3 in, 3 out]
  n272 = Match Pattern(string=w14, regular expression="\\[Dev\\]") -> (before substring=w11:string, after substring=w12:string)  [unwired: 1 in, 2 out]
  n273 = local write "Dev Notes"(w12) -> ()
  n274 = local write "notes"(w11) -> ()
  n275 = Match First String(2:w37, 3:w36) -> (0:w35:i32)  [unwired: 1 out]
  n276 = Bundle("value"=w41, "value"=w40, "index"=w35) -> (w29:cluster{"value":i32, "value":i32, "index":i32})  [unwired: 1 out]
  n277 = while {
    tunnel: w15 -> [w437]
    stop <- FALSE stop-if-true
    n278 = local read "Dev Notes"() -> (w441:string)
    n279 = local read "notes"() -> (w436:string)
    n280 = feedback #1() -> (w435:string)  [unwired: 1 in]
    n281 = feedback-in #1(w441) -> ()
    n282 = feedback-in #2(w436) -> ()
    n283 = feedback #2() -> (w442:string)  [unwired: 1 in]
    n284 = Not Equal?(x=w441, y=w435) -> (x != y?=w439:bool)
    n285 = Not Equal?(x=w436, y=w442) -> (x != y?=w440:bool)
    n286 = Or(x=w440, y=w439) -> (x .or. y?=w438:bool)
    n287 = Wait (ms)(milliseconds to wait=1000) -> ()  [unwired: 1 out]
    n288 = case shown="True" w438 {
      tunnel: w437 -> [_ w449]
      tunnel: w436 -> [_ w447]
      tunnel: w435 -> [_ w446]
      frame False {
      }
      frame True {
        n289 = Concatenate Strings(w447, "[Dev]", w446) -> (w448:string)
        n290 = Write to Text File(file (use dialog)=w449, text=w448) -> ()  [unwired: 2 in, 3 out]
      }
    }
  }
  n291 = property on="On/Off" class="Bool (strict)"("Visible"=w52) -> ()  [unwired: 2 in, 2 out]
  n292 = property on="Motor" class="Clust (strict)"("Visible"=w52) -> ()  [unwired: 2 in, 2 out]
  n293 = property on="Progress" class="Clust (strict)"("Visible"=w52) -> ()  [unwired: 2 in, 2 out]
  n294 = property on="Ring" class="Ring (strict)"("Visible"=w52) -> ()  [unwired: 2 in, 2 out]
  n295 = property on="Camera Settings" class="Clust (strict)"("Val(Sgnl)"=w29) -> ()  [unwired: 2 in, 2 out]
  n296 = property on="Rev/Fwd" class="Clust (strict)"("Visible"=w52) -> ()  [unwired: 2 in, 2 out]
  n297 = property on="Camera Settings" class="Clust (strict)"("Visible"=w52) -> ()  [unwired: 2 in, 2 out]
  n298 = local write "DB Camera Config"(w52) -> ()
  "MotorName2" <- "Right Drive Motor"
  "MotorName1" <- "Left Drive Motor"
  "MotorName4" <- ""
  "MotorName3" <- "Arm Motor"
